vi "Application Main.vi"() -> ()   [LabVIEW 2020]
doc: "The main launcher application for the MGI Monitored Actor Example.\n\nCopyright (c) 2010, Moore Good Ideas, Inc.\n\nAll rights reserved.\n\nRedistribution and use in source and binary forms, with or without modification, are permitted provided that the following conditions are met:\n\n * Redistributions of source code must retain the above copyright notice, this list of conditions and the following disclaimer.\n * Redistributions in binary form must reproduce the above copyright notice, this list of conditions and the following disclaimer in the documentation and/or other materials provided with the distribution.\n * Neither the name of Moore Good Ideas, Inc. nor the names of its contributors may be used to endorse or promote products derived from this software without specific prior written permission.\n\nTHIS SOFTWARE IS PROVIDED BY THE COPYRIGHT HOLDERS AND CONTRIBUTORS \"AS IS\" AND ANY EXPRESS OR IMPLIED WARRANTIES, INCLUDING, BUT NOT LIMITED TO, THE IMPLIED WARRANTIES OF MERCHANTABILITY AND FITNESS FOR A PARTICULAR PURPOSE ARE DISCLAIMED. IN NO EVENT SHALL THE COPYRIGHT OWNER OR CONTRIBUTORS BE LIABLE FOR ANY DIRECT, INDIRECT, INCIDENTAL, SPECIAL, EXEMPLARY, OR CONSEQUENTIAL DAMAGES (INCLUDING, BUT NOT LIMITED TO, PROCUREMENT OF SUBSTITUTE GOODS OR SERVICES; LOSS OF USE, DATA, OR PROFITS; OR BUSINESS INTERRUPTION) HOWEVER CAUSED AND ON ANY THEORY OF LIABILITY, WHETHER IN CONTRACT, STRICT LIABILITY, OR TORT (INCLUDING NEGLIGENCE OR OTHERWISE) ARISING IN ANY WAY OUT OF THE USE OF THIS SOFTWARE, EVEN IF ADVISED OF THE POSSIBILITY OF SUCH DAMAGE."
uses:
  Special Monitor/Special Monitor.lvclass
  C:/Program Files/National Instruments/LabVIEW 2020/vi.lib/MGI/Monitored Actor/Actor Monitor/Actor Monitor/Actor Monitor.lvclass
  <vilib>/MGI/Monitored Actor/Monitored Actor.lvlib
  Example Actor/Example Actor/Example Actor.lvclass
  <vilib>/MGI/Monitored Actor/Actor Monitor/Actor Monitor/Actor Monitor.lvclass
panel:
  in  "Use Special Monitor?":bool
  in  "Actors/Level":i32=2
  in  "Levels to Spawn":i32=2
  # "Levels to Spawn will set the depth for how many levels of spawned actors to instantiate.\nActors/Level will set the number of nested actors for each spawned level.\n\nSelect values for Levels to Spawn and Actors/Level, then run this VI to see the spawned Actors\nin the Actor Monitor.\n\nYou will need to use the features of the Actor Monitor window to stop the actors.\n\nSeleting \"Use Special Monitor\" will use a user-defined monitor to show how a user could override the monitor interface if desired."
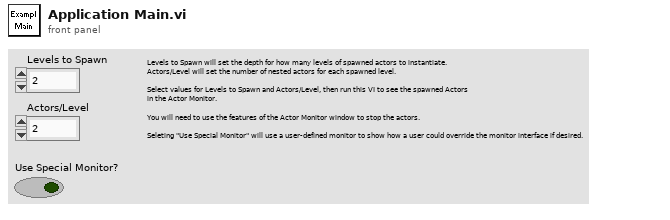
[diagram p1: front panel]
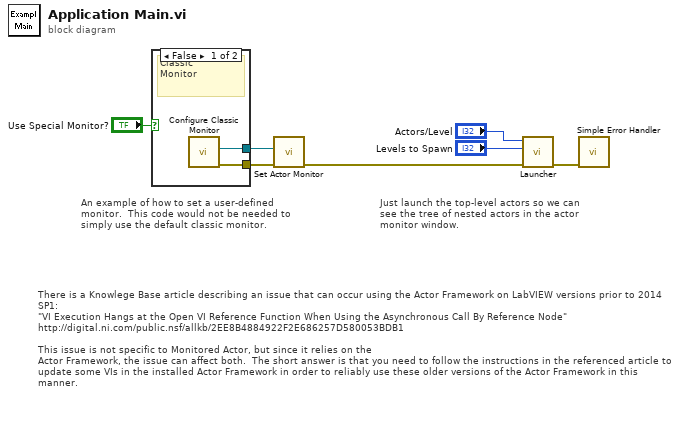
[diagram p0: block diagram]
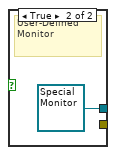
[diagram p2: hidden frame]
diagram:
  # "Just launch the top-level actors so we can\nsee the tree of nested actors in the actor monitor window."
  # "An example of how to set a user-defined monitor.  This code would not be needed to simply use the default classic monitor."
  # "There is a Knowlege Base article describing an issue that can occur using the Actor Framework on LabVIEW versions prior to 2014 SP1:\n\"VI Execution Hangs at the Open VI Reference Function When Using the Asynchronous Call By Reference Node\"\nhttp://digital.ni.com/public.nsf/allkb/2EE8B4884922F2E686257D580053BDB1\n\nThis issue is not specific to Monitored Actor, but since it relies on the\nActor Framework, the issue can affect both.  The short answer is that you need to follow the instructions in the referenced article to update some VIs in the installed Actor Framework in order to reliably use these older versions of the Actor Framework in this manner."
  n1 = case shown="False" "Use Special Monitor?" {
    tunnel: [w9 _] -> w7
    tunnel: [w8 refnum<class "Special Monitor.lvclass"> refnum ("Special Monitor.lvclass")] -> w6
    frame False {
      # "Classic \nMonitor"
      n2 = call <vilib>:"Configure Classic Monitor.vi"() -> ("error out"=w9:errorcluster, "Classic Monitor out"=w8:refnum<class "Actor Monitor.lvclass">)  [unwired: 10 in]
    }
    frame True {
      # "User-Defined\nMonitor"
    }
  }
  n3 = call <vilib>:"Set Actor Monitor.vi"("error in (no error)"=w7, "Actor Monitor"=w6) -> ("error out"=w4:errorcluster)  [unwired: 9 in]
  n4 = call "Launcher.vi"("error in (no error)"=w4, "Levels to Spawn"="Levels to Spawn", "Actors/Level"="Actors/Level") -> ("error out"=w3:errorcluster)  [unwired: 8 in]
  n5 = call <vilib>:"Simple Error Handler.vi"("error in (no error)"=w3) -> ()  [unwired: 4 in, 5 out]
